vi "fpga_Wait Function.vi"(2 "start? (F)":bool, 7 "timeout (ms)":u32) -> (8 "timeout?":bool)   [LabVIEW 2012, in "NI_EP_Protection_FPGA.lvlib"]
uses:
  <vilib>/addons/Electrical Power/Protection/NI_EP_Protection_FPGA.lvlib
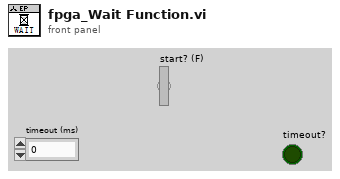
[diagram p1: front panel]
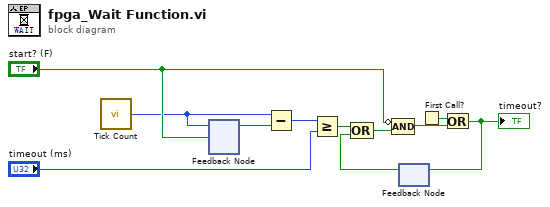
[diagram p0: block diagram]
diagram:
  n1 = call "Tick Count"() -> ("Tick Count(mSec)"=w6:u32)
  n2 = feedback #1() -> (w11:u32)  [unwired: 1 in]
  n3 = feedback-in #1(w6, "start? (F)") -> ()
  n4 = Subtract(x=w6, y=w11) -> (x-y=w10:u32)
  n5 = Greater Or Equal?(x=w10, y="timeout (ms)") -> (x >= y?=w2:bool)
  n6 = feedback #2() -> (w1:bool)  [unwired: 1 in]
  n7 = Compound Arithmetic op=OR(w2, w1) -> (w8:bool)
  n8 = Compound Arithmetic op=AND(invert "start? (F)", w8) -> (w4:bool)
  n9 = First Call?() -> (First Call?: T/F=w5:bool)
  n10 = Or(x=w5, y=w4) -> (x .or. y?=w3:bool)
  "timeout?" <- w3
  n11 = feedback-in #2(w3) -> ()
